vi "fromCluster.vi"(8 "error in (no error)":errorcluster, 10 "ACNET Device Cluster":T1, 11 "ACNET Device in":refnum<class "Copy of ACNET Device.lvclass">) -> (0 "error out":errorcluster, 3 "ACNET Device out":refnum<class "Copy of ACNET Device.lvclass">)   [LabVIEW 2013, in "Copy of ACNET Device.lvclass"]
uses:
  Copy of ACNET Device.lvclass
  Copy of ACNET Device.lvclass/Copy of ACNET Device.ctl
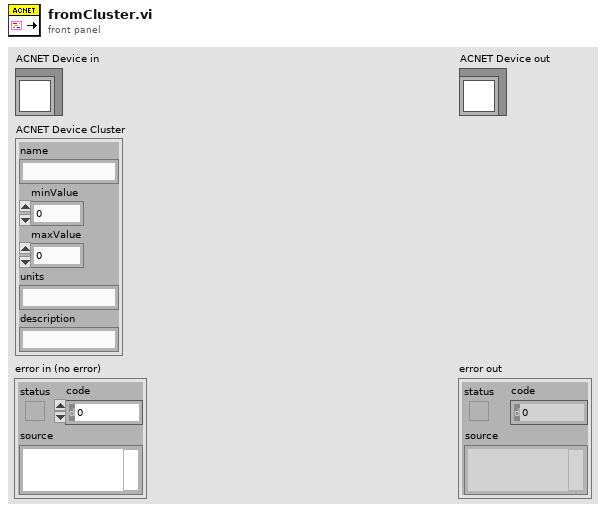
[diagram p1: front panel]
types:
  T1 = cluster{"name":string, "minValue":dbl, "maxValue":dbl, "units":string, "description":string}
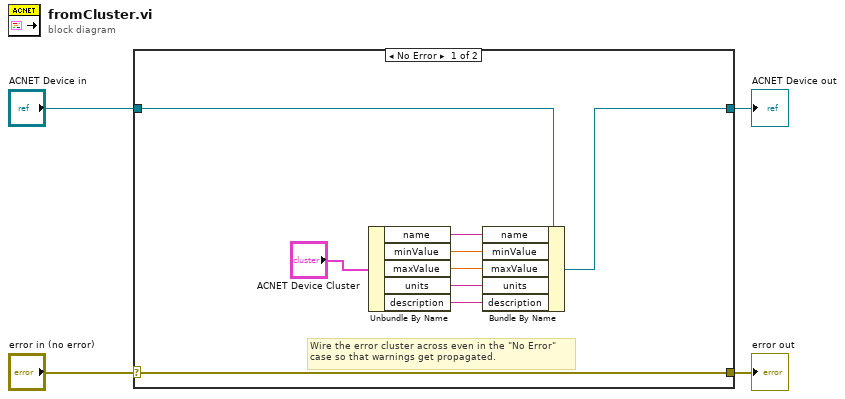
[diagram p0: block diagram]
diagram:
  n1 = case shown="No Error" "error in (no error)" {
    selector: "error in (no error)" -> [w6 w15]
    tunnel: [w6 w15] -> w3
    tunnel: [w7 w14] -> w1
    tunnel: "ACNET Device in" -> [w8 w14]
    frame No Error {
      # "Wire the error cluster across even in the \"No Error\"\ncase so that warnings get propagated."
      n2 = Unbundle By Name("ACNET Device Cluster") -> ("name"=w13:string, "minValue"=w12:dbl, "maxValue"=w11:dbl, "units"=w10:string, "description"=w5:string)
      n3 = Bundle By Name(cluster=w8, "name"=w13, "minValue"=w12, "maxValue"=w11, "units"=w10, "description"=w5) -> (w7:refnum<class "Copy of ACNET Device.lvclass">)
    }
    frame Error {
    }
  }
  "error out" <- w3
  "ACNET Device out" <- w1
